vi "Shift Master.vi"(8 "error in (no error)":errorcluster) -> (0 "error out":errorcluster)   [LabVIEW 2017]
uses:
  <vilib>/Utility/miscctls.llb/LVRowAndColumnTypeDef.ctl
  <vilib>/Utility/miscctls.llb/LVBoundsTypeDef.ctl
  <vilib>/addons/database/Connection.llb/DB Tools Open Connec (Path).vi
  Globle/Current date.vi
  <vilib>/addons/database/NI_Database_API.lvlib
panel:
  in  "Back 2":bool
  in  "UPDATE   2":bool
  in  "MANUALLY":bool
  in  "12 HR SHIFT IN 24 HR FORMATE":bool
  in  "8 HR SHIFT IN 24 HR FORMATE":bool
  in  "Shift 3 Stop Time":timestamp format="%<%H-%M-%S>T"
  in  "Shift 2Stop Time":timestamp format="%<%H:%M:%S>T"
  in  "Shift 3 Start Time":timestamp format="%<%H-%M-%S>T"
  in  "Shift 2 Start Time":timestamp format="%<%H:%M:%S>T"
  in  "Shift 1 Stop Time":timestamp=timestamp(-9561628800 s since 1904-01-01) format="%<%H:%M:%S>T"
  in  "Shift 1 Start time":timestamp=timestamp(-9561628800 s since 1904-01-01) format="%<%H:%M:%S>T"
  # "Shift Master"
  # "Shift Start Time"
  # "Shift End Time"
  # "Shift Name"
  # "Shift One"
  # "Shift Two"
  # "Shift Three"
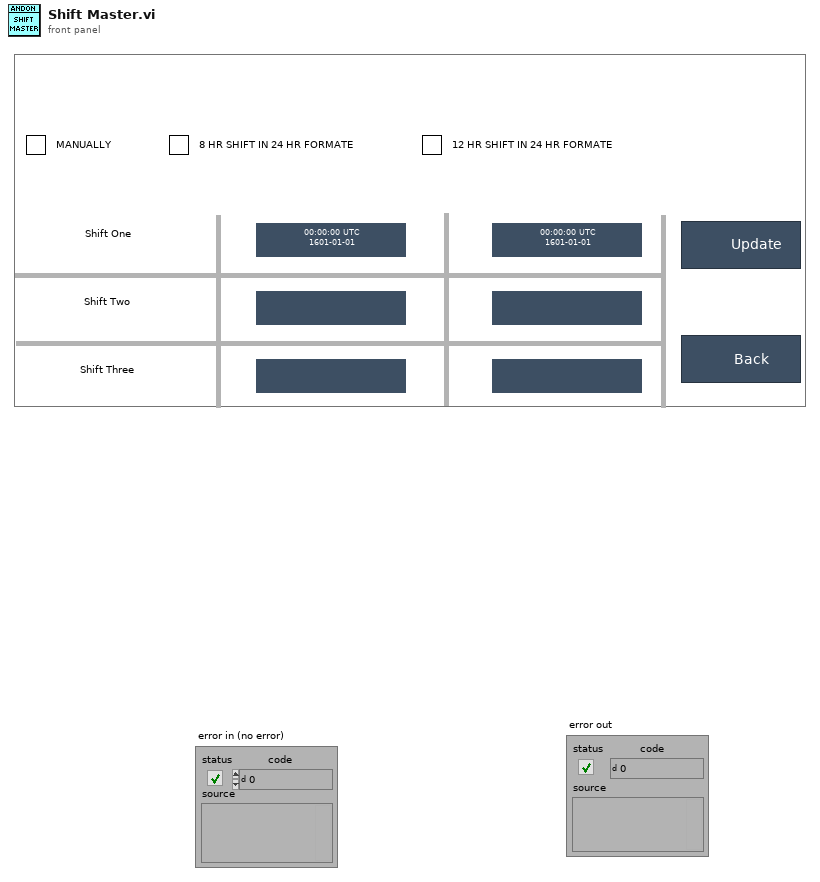
[diagram p1: front panel]
types:
  T1 = typedef "LVBoundsTypeDef.ctl" = cluster{"Width":u32, "Height":u32}
  T2 = typedef "LVRowAndColumnTypeDef.ctl" = cluster{"Row":i32, "Column":i32}
  T3 = enum8{"Enabled", "Disabled", "Disabled and Grayed Out"}
  T4 = typedef "NI_Database_API.lvlib/Conn ObjectReference.ctl" = refnum<k1>
  T5 = cluster{"Shift 3 Start Time":timestamp, "Shift 3 Stop Time ":timestamp}
  T6 = cluster{"Shift 2 Start Time":timestamp, "Shift 2Stop Time":timestamp}
  T7 = cluster{"Shift 1 Start time":timestamp, "Shift 1 Stop Time":timestamp}
  T8 = cluster{"Shift 3 Start Time":timestamp, "Shift 3 Stop Time ":timestamp}[]
  T9 = enum32{"invalid app kind", "Development System", "Run Time System", "Student Edition", "Embedded LabVIEW", "Evaluation", "Custom"}
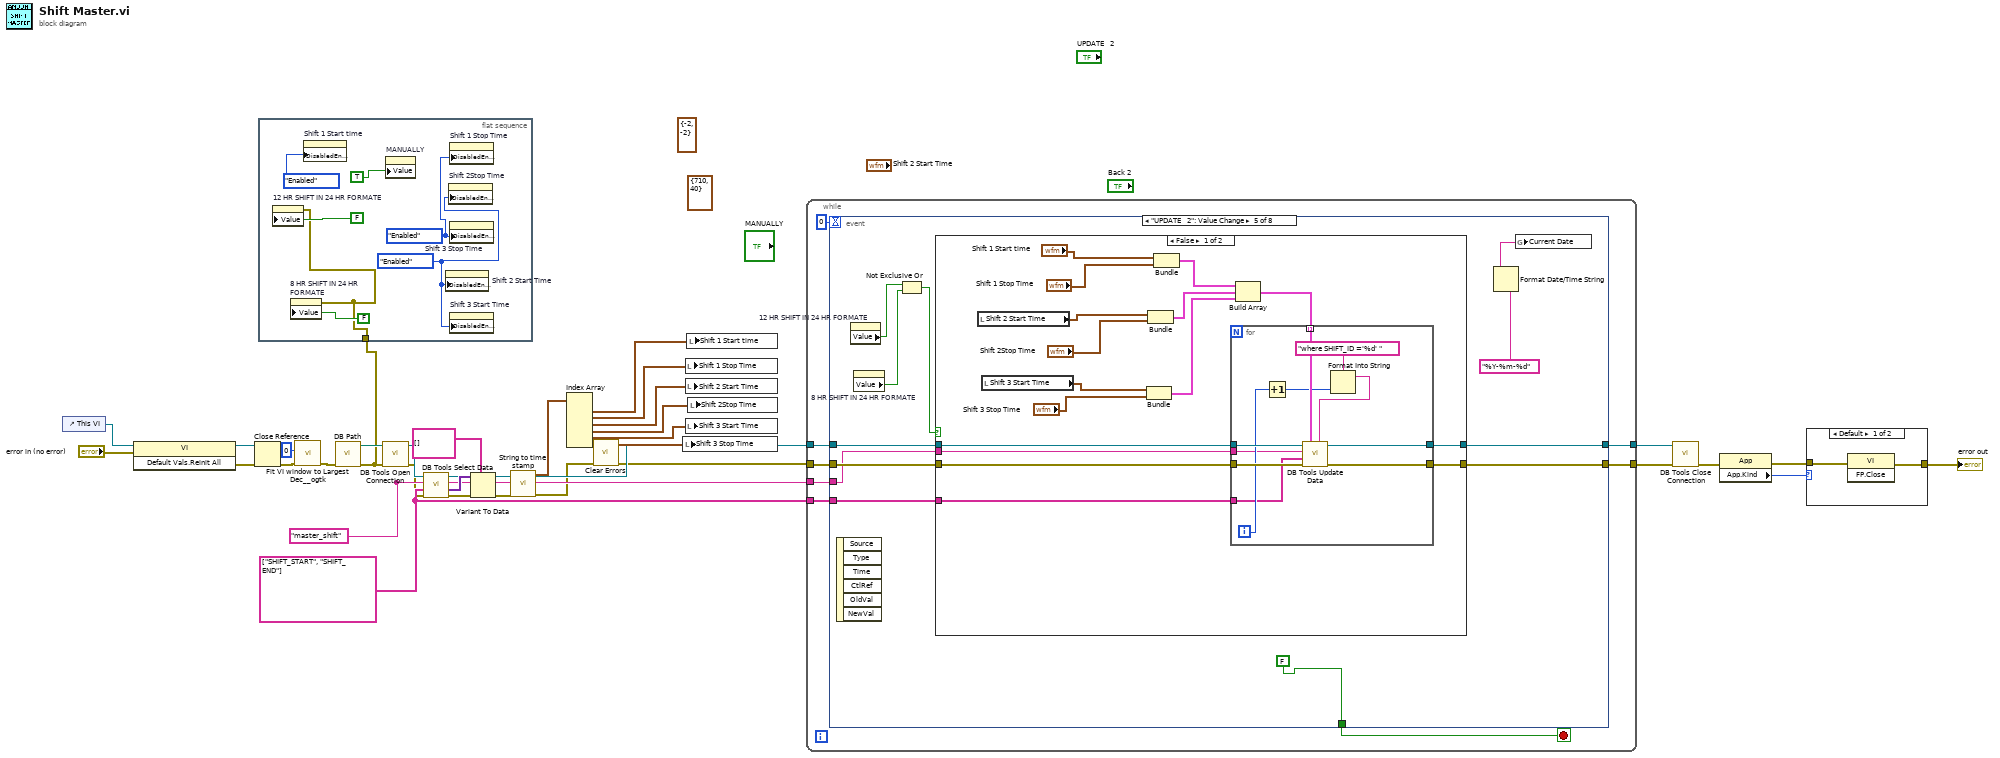
[diagram p0: block diagram]
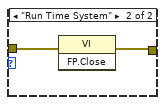
[diagram p2: hidden frame]
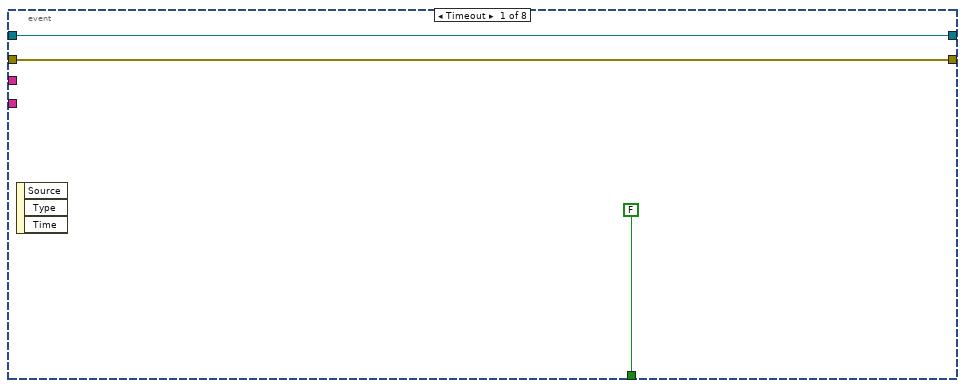
[diagram p3: hidden frame]
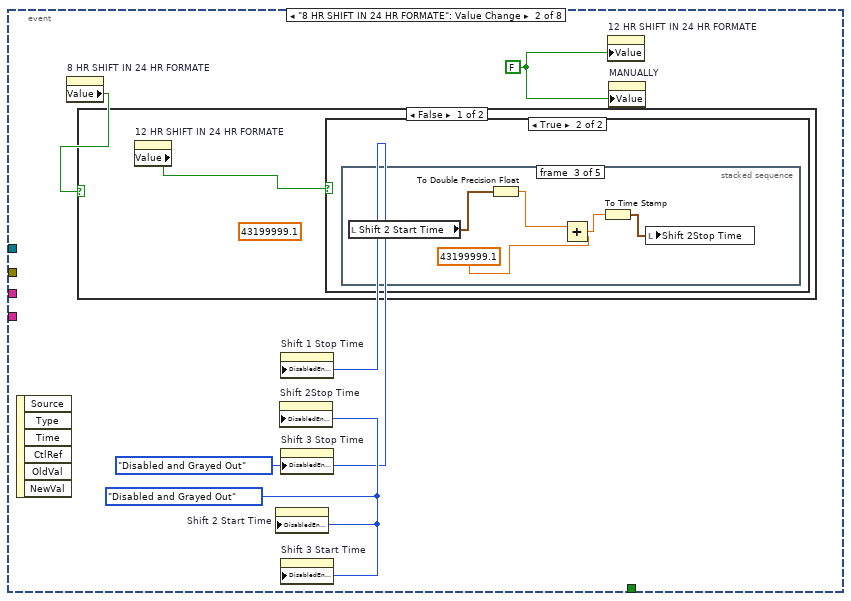
[diagram p4: hidden frame]
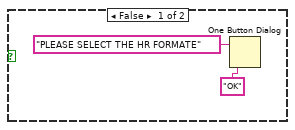
[diagram p5: hidden frame]
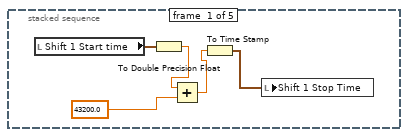
[diagram p6: hidden frame]
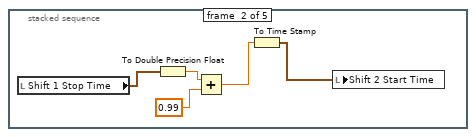
[diagram p7: hidden frame]
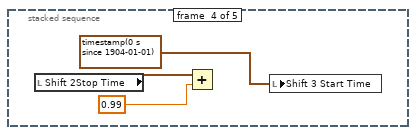
[diagram p8: hidden frame]
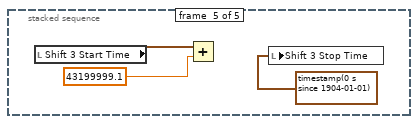
[diagram p9: hidden frame]
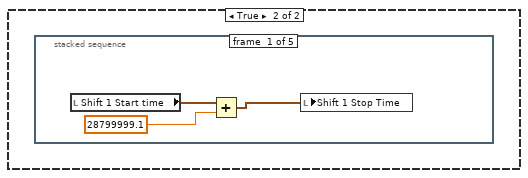
[diagram p10: hidden frame]
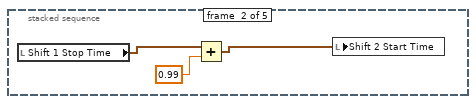
[diagram p11: hidden frame]
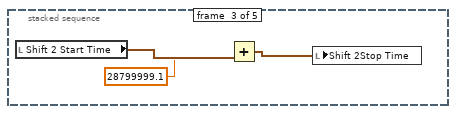
[diagram p12: hidden frame]
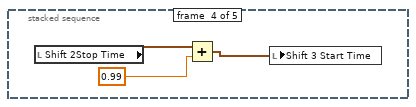
[diagram p13: hidden frame]
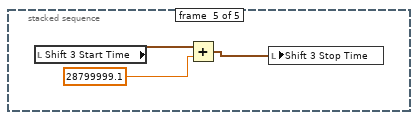
[diagram p14: hidden frame]
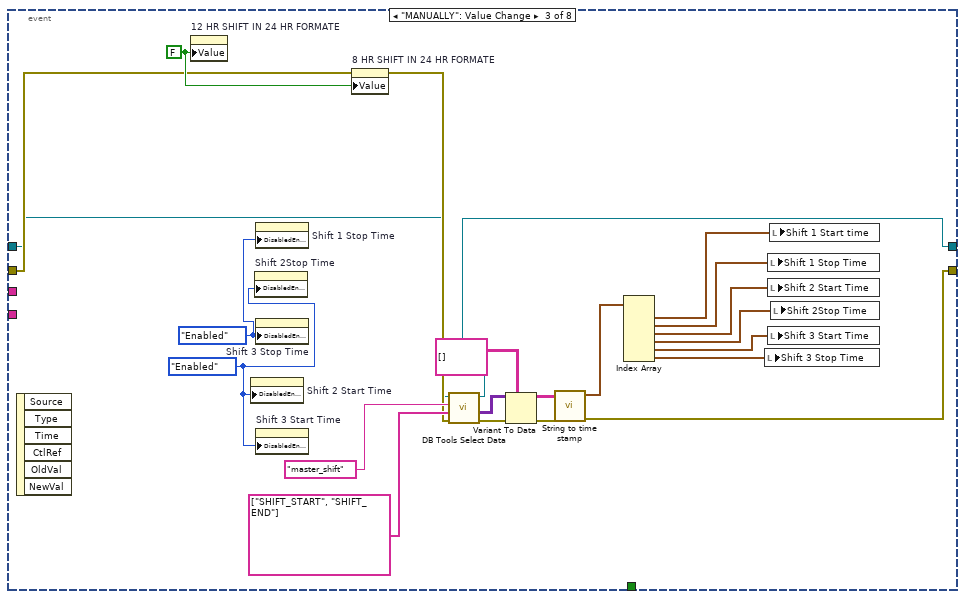
[diagram p15: hidden frame]
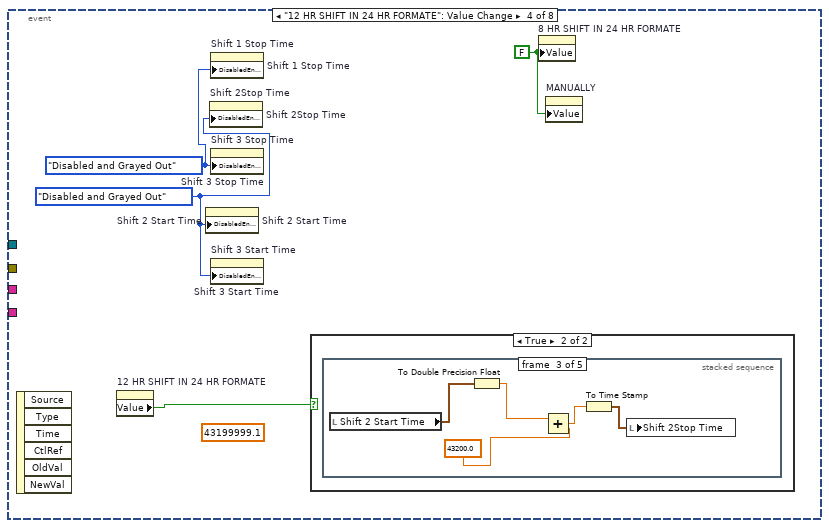
[diagram p16: hidden frame]
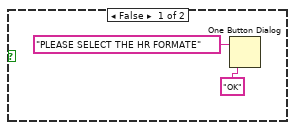
[diagram p17: hidden frame]
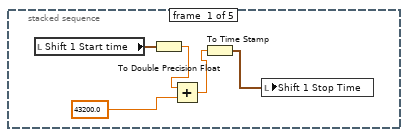
[diagram p18: hidden frame]
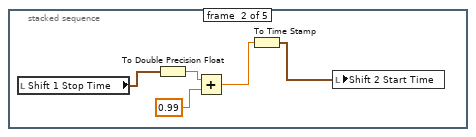
[diagram p19: hidden frame]
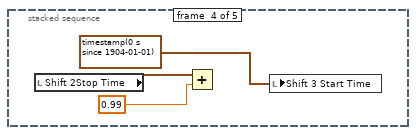
[diagram p20: hidden frame]
diagram:
  w10 = string[] ["SHIFT_START", "SHIFT_END"] ("columns")
  w11 = "master_shift" ("table")
  (unwired) T1 {"Width"=710, "Height"=40} ("Active Cell:Cell Size")
  (unwired) T2 {"Row"=-2, "Column"=-2} ("Active Cell:Active Cell")
  n1 = control-ref of="This VI"() -> (w34:refnum<vi>)
  n2 = invoke class="VI" method="Default Vals.Reinit All"(reference=w34, error in="error in (no error)") -> (reference out=w31:refnum<vi>, error out=w32:errorcluster)  [unwired: 1 in, 1 out]
  n3 = Close Reference(reference=w31, error in (no error)=w32) -> (error out=w4:errorcluster)
  n4 = flat-sequence {
    tunnel: w1 -> [w36]
    frame #0 {
      w41 = T3."Enabled" ("Disabled")
      w40 = T3."Enabled" ("Disabled")
      n5 = property on="12 HR SHIFT IN 24 HR FORMATE" class="Bool (strict)"(error in=w36, "Value"=FALSE ("12 HR FORMATE")) -> ()  [unwired: 1 in, 2 out]
      n6 = property on="8 HR SHIFT IN 24 HR FORMATE" class="Bool (strict)"(error in=w36, "Value"=FALSE ("8 HR FORMATE")) -> ()  [unwired: 1 in, 2 out]
      n7 = property on="Shift 1 Start time" class="AbsTime (strict)"("DisabledEnum"=T3."Enabled" ("Disabled")) -> ()  [unwired: 2 in, 2 out]
      n8 = property on="MANUALLY" class="Bool (strict)"("Value"=TRUE ("12 HR FORMATE")) -> ()  [unwired: 2 in, 2 out]
      n9 = property on="Shift 2 Start Time" class="AbsTime (strict)"("DisabledEnum"=w41) -> ()  [unwired: 2 in, 2 out]
      n10 = property on="Shift 2Stop Time" class="AbsTime (strict)"("DisabledEnum"=w41) -> ()  [unwired: 2 in, 2 out]
      n11 = property on="Shift 1 Stop Time" class="AbsTime (strict)"("DisabledEnum"=w40) -> ()  [unwired: 2 in, 2 out]
      n12 = property on="Shift 3 Stop Time" class="AbsTime (strict)"("DisabledEnum"=w40) -> ()  [unwired: 2 in, 2 out]
      n13 = property on="Shift 3 Start Time" class="AbsTime (strict)"("DisabledEnum"=w41) -> ()  [unwired: 2 in, 2 out]
    }
  }
  n14 = call <userlib>:"Fit VI window to Largest Dec__ogtk.vi"("error in (no error)"=w4, "border spacing (2 px)"=0) -> ("error out"=w3:errorcluster)  [unwired: 4 in, 1 out]
  n15 = call "DB Path.vi"("error in"=w3) -> ("error out"=w1:errorcluster, "DB Path"=w27:path)  [unwired: 9 in]
  n16 = call-poly <vilib>:"DB Tools Open Connection.vi"("error in (no error)"=w1, "connection information"=w27) -> ("error out"=w5:errorcluster, "connection reference"=w6:T4)  [unwired: 6 in]
  n17 = call <vilib>:"DB Tools Select Data.vi"("error in (no error)"=w5, "columns"=w10, "table"=w11, "connection reference"=w6) -> ("error out"=w25:errorcluster, "data"=w26:variant[][], "connection reference out"=w15:T4)  [unwired: 2 in]
  n18 = Variant To Data(error in=w25, type=string[][] [], Variant=w26) -> (data=w9:string[][], error out=w23:errorcluster)
  n19 = call "String to time stamp.vi"("error in (no error)"=w23, "Data In"=w9) -> ("error out"=w8:errorcluster, "Time Stamp Out"=w22:timestamp[])  [unwired: 8 in]
  n20 = Index Array(array=w22) -> (element #1=w21:timestamp, element #2=w20:timestamp, element #3=w19:timestamp, element #4=w18:timestamp, element #5=w17:timestamp, element #6=w16:timestamp)  [unwired: 6 in]
  n21 = call <vilib>:"Clear Errors.vi"("error in (no error)"=w8) -> ("error out"=w7:errorcluster)  [unwired: 5 in, 1 out]
  n22 = local write "Shift 3 Stop Time"(w16) -> ()
  n23 = local write "Shift 1 Stop Time"(w20) -> ()
  n24 = local write "Shift 2 Start Time"(w19) -> ()
  n25 = local write "Shift 3 Start Time"(w17) -> ()
  n26 = local write "Shift 1 Start time"(w21) -> ()
  n27 = local write "Shift 2Stop Time"(w18) -> ()
  n28 = while {
    tunnel: w7 -> [w49]
    tunnel: [w47] -> w14
    tunnel: w15 -> [w46]
    tunnel: [w45] -> w12
    tunnel: w11 -> [w44]
    tunnel: w10 -> [w43]
    stop <- w48 stop-if-true
    n29 = event shown="[4] \"UPDATE   2\": Value Change" {
      selector: _ -> [_ _ _ _ _ _ _ _]
      dyn-events: _ -> [_ _ _ _ _ _ _ _]
      timeout: 0 -> [_ _ _ _ _ _ _ _]
      tunnel: w49 -> [w51 _ w99 _ w158 w191 w193 w200]
      tunnel: [FALSE _ _ _ FALSE TRUE _ FALSE] -> w48
      tunnel: [w51 _ w98 _ w154 w191 w193 w200] -> w47
      tunnel: w46 -> [w52 _ w97 _ w157 w192 _ w198]
      tunnel: [w52 _ w96 _ w153 w192 _ w198] -> w45
      tunnel: w44 -> [_ _ _ _ w156 _ _ _]
      tunnel: w43 -> [_ _ _ _ w155 _ _ _]
      event Timeout {
        n30 = event-data() -> ()  [unwired: 1 in, 3 out]
      }
      event "8 HR SHIFT IN 24 HR FORMATE": Value Change {
        w54 = T3."Disabled and Grayed Out" ("Disabled")
        w53 = T3."Disabled and Grayed Out" ("Disabled")
        w55 = FALSE ("12 HR FORMATE")
        n31 = event-data() -> ()  [unwired: 1 in, 6 out]
        n32 = property on="8 HR SHIFT IN 24 HR FORMATE" class="Bool (strict)"() -> ("Value"=w56:bool)  [unwired: 2 in, 2 out]
        n33 = case shown="False" w56 {
          frame False {
            (unwired) 43199999.1 ("y")
            n34 = property on="12 HR SHIFT IN 24 HR FORMATE" class="Bool (strict)"() -> ("Value"=w57:bool)  [unwired: 2 in, 2 out]
            n35 = case shown="True" w57 {
              frame False {
                n36 = One Button Dialog(message="PLEASE SELECT THE HR FORMATE", button name ("OK")="OK") -> ()  [unwired: 1 out]
              }
              frame True {
                n37 = stacked-sequence {
                  frame #0 {
                    n38 = local read "Shift 1 Start time"() -> (w63:timestamp)
                    n39 = To Double Precision Float(number=w63) -> (double precision float=w62:dbl)
                    n40 = Add(x=w62, y=43200.0) -> (x+y=w61:dbl)
                    n41 = To Time Stamp(1:w61) -> (0:w60:timestamp)
                    n42 = local write "Shift 1 Stop Time"(w60) -> ()
                  }
                  frame #1 {
                    n43 = local read "Shift 1 Stop Time"() -> (w66:timestamp)
                    n44 = To Double Precision Float(number=w66) -> (double precision float=w65:dbl)
                    n45 = Add(x=w65, y=0.99) -> (x+y=w67:dbl)
                    n46 = To Time Stamp(1:w67) -> (0:w68:timestamp)
                    n47 = local write "Shift 2 Start Time"(w68) -> ()
                  }
                  frame #2 {
                    n48 = local read "Shift 2 Start Time"() -> (w71:timestamp)
                    n49 = To Double Precision Float(number=w71) -> (double precision float=w70:dbl)
                    n50 = Add(x=w70, y=43199999.1) -> (x+y=w73:dbl)
                    n51 = To Time Stamp(1:w73) -> (0:w72:timestamp)
                    n52 = local write "Shift 2Stop Time"(w72) -> ()
                  }
                  frame #3 {
                    n53 = local read "Shift 2Stop Time"() -> (w77:timestamp)
                    n54 = Add(x=w77, y=0.99) -> ()  [unwired: 1 out]
                    n55 = local write "Shift 3 Start Time"(timestamp(0 s since 1904-01-01) ("x+y")) -> ()
                  }
                  frame #4 {
                    n56 = local read "Shift 3 Start Time"() -> (w80:timestamp)
                    n57 = Add(x=w80, y=43199999.1) -> ()  [unwired: 1 out]
                    n58 = local write "Shift 3 Stop Time"(timestamp(0 s since 1904-01-01) ("x+y")) -> ()
                  }
                }
              }
            }
          }
          frame True {
            n59 = stacked-sequence {
              frame #0 {
                n60 = local read "Shift 1 Start time"() -> (w83:timestamp)
                n61 = Add(x=w83, y=28799999.1) -> (x+y=w81:timestamp)
                n62 = local write "Shift 1 Stop Time"(w81) -> ()
              }
              frame #1 {
                n63 = local read "Shift 1 Stop Time"() -> (w84:timestamp)
                n64 = Add(x=w84, y=0.99) -> (x+y=w86:timestamp)
                n65 = local write "Shift 2 Start Time"(w86) -> ()
              }
              frame #2 {
                n66 = local read "Shift 2 Start Time"() -> (w89:timestamp)
                n67 = Add(x=w89, y=28799999.1) -> (x+y=w88:timestamp)
                n68 = local write "Shift 2Stop Time"(w88) -> ()
              }
              frame #3 {
                n69 = local read "Shift 2Stop Time"() -> (w91:timestamp)
                n70 = Add(x=w91, y=0.99) -> (x+y=w92:timestamp)
                n71 = local write "Shift 3 Start Time"(w92) -> ()
              }
              frame #4 {
                n72 = local read "Shift 3 Start Time"() -> (w95:timestamp)
                n73 = Add(x=w95, y=28799999.1) -> (x+y=w94:timestamp)
                n74 = local write "Shift 3 Stop Time"(w94) -> ()
              }
            }
          }
        }
        n75 = property on="Shift 2 Start Time" class="AbsTime (strict)"("DisabledEnum"=w54) -> ()  [unwired: 2 in, 2 out]
        n76 = property on="Shift 2Stop Time" class="AbsTime (strict)"("DisabledEnum"=w54) -> ()  [unwired: 2 in, 2 out]
        n77 = property on="Shift 1 Stop Time" class="AbsTime (strict)"("DisabledEnum"=w53) -> ()  [unwired: 2 in, 2 out]
        n78 = property on="Shift 3 Stop Time" class="AbsTime (strict)"("DisabledEnum"=w53) -> ()  [unwired: 2 in, 2 out]
        n79 = property on="Shift 3 Start Time" class="AbsTime (strict)"("DisabledEnum"=w54) -> ()  [unwired: 2 in, 2 out]
        n80 = property on="12 HR SHIFT IN 24 HR FORMATE" class="Bool (strict)"("Value"=w55) -> ()  [unwired: 2 in, 2 out]
        n81 = property on="MANUALLY" class="Bool (strict)"("Value"=w55) -> ()  [unwired: 2 in, 2 out]
      }
      event "MANUALLY": Value Change {
        w115 = FALSE ("12 HR SHIFT IN 24 HR FORMATE")
        w117 = T3."Enabled" ("Disabled")
        w116 = T3."Enabled" ("Disabled")
        n82 = event-data() -> ()  [unwired: 1 in, 6 out]
        n83 = property on="12 HR SHIFT IN 24 HR FORMATE" class="Bool (strict)"("Value"=w115) -> ()  [unwired: 2 in, 2 out]
        n84 = property on="Shift 2 Start Time" class="AbsTime (strict)"("DisabledEnum"=w117) -> ()  [unwired: 2 in, 2 out]
        n85 = property on="Shift 2Stop Time" class="AbsTime (strict)"("DisabledEnum"=w117) -> ()  [unwired: 2 in, 2 out]
        n86 = property on="Shift 1 Stop Time" class="AbsTime (strict)"("DisabledEnum"=w116) -> ()  [unwired: 2 in, 2 out]
        n87 = property on="Shift 3 Stop Time" class="AbsTime (strict)"("DisabledEnum"=w116) -> ()  [unwired: 2 in, 2 out]
        n88 = property on="Shift 3 Start Time" class="AbsTime (strict)"("DisabledEnum"=w117) -> ()  [unwired: 2 in, 2 out]
        n89 = property on="8 HR SHIFT IN 24 HR FORMATE" class="Bool (strict)"(error in=w99, "Value"=w115) -> (error out=w100:errorcluster)  [unwired: 1 in, 1 out]
        n90 = call <vilib>:"DB Tools Select Data.vi"("error in (no error)"=w100, "columns"=string[] ["SHIFT_START", "SHIFT_END"], "table"="master_shift", "connection reference"=w97) -> ("error out"=w113:errorcluster, "data"=w114:variant[][], "connection reference out"=w96:T4)  [unwired: 2 in]
        n91 = Variant To Data(error in=w113, type=string[][] [], Variant=w114) -> (data=w104:string[][], error out=w112:errorcluster)
        n92 = call "String to time stamp.vi"("error in (no error)"=w112, "Data In"=w104) -> ("error out"=w98:errorcluster, "Time Stamp Out"=w111:timestamp[])  [unwired: 8 in]
        n93 = Index Array(array=w111) -> (element #1=w110:timestamp, element #2=w109:timestamp, element #3=w108:timestamp, element #4=w107:timestamp, element #5=w106:timestamp, element #6=w105:timestamp)  [unwired: 6 in]
        n94 = local write "Shift 3 Stop Time"(w105) -> ()
        n95 = local write "Shift 1 Stop Time"(w109) -> ()
        n96 = local write "Shift 2 Start Time"(w108) -> ()
        n97 = local write "Shift 3 Start Time"(w106) -> ()
        n98 = local write "Shift 1 Start time"(w110) -> ()
        n99 = local write "Shift 2Stop Time"(w107) -> ()
      }
      event "12 HR SHIFT IN 24 HR FORMATE": Value Change {
        w119 = T3."Disabled and Grayed Out" ("Disabled")
        w118 = T3."Disabled and Grayed Out" ("Disabled")
        w120 = T3."Disabled and Grayed Out" ("Disabled")
        w121 = T3."Disabled and Grayed Out" ("Disabled")
        (unwired) 43199999.1 ("y")
        w122 = FALSE ("8 HR FORMATE")
        n100 = event-data() -> ()  [unwired: 1 in, 6 out]
        n101 = property on="12 HR SHIFT IN 24 HR FORMATE" class="Bool (strict)"() -> ("Value"=w123:bool)  [unwired: 2 in, 2 out]
        n102 = property on="Shift 2 Start Time" class="AbsTime (strict)"("DisabledEnum"=w119) -> ()  [unwired: 2 in, 2 out]
        n103 = property on="Shift 2 Start Time" class="AbsTime (strict)"("DisabledEnum"=w120) -> ()  [unwired: 2 in, 2 out]
        n104 = property on="Shift 2Stop Time" class="AbsTime (strict)"("DisabledEnum"=w119) -> ()  [unwired: 2 in, 2 out]
        n105 = property on="Shift 2Stop Time" class="AbsTime (strict)"("DisabledEnum"=w120) -> ()  [unwired: 2 in, 2 out]
        n106 = property on="Shift 1 Stop Time" class="AbsTime (strict)"("DisabledEnum"=w118) -> ()  [unwired: 2 in, 2 out]
        n107 = property on="Shift 1 Stop Time" class="AbsTime (strict)"("DisabledEnum"=w121) -> ()  [unwired: 2 in, 2 out]
        n108 = property on="Shift 3 Stop Time" class="AbsTime (strict)"("DisabledEnum"=w118) -> ()  [unwired: 2 in, 2 out]
        n109 = property on="Shift 3 Stop Time" class="AbsTime (strict)"("DisabledEnum"=w121) -> ()  [unwired: 2 in, 2 out]
        n110 = property on="Shift 3 Start Time" class="AbsTime (strict)"("DisabledEnum"=w119) -> ()  [unwired: 2 in, 2 out]
        n111 = property on="Shift 3 Start Time" class="AbsTime (strict)"("DisabledEnum"=w120) -> ()  [unwired: 2 in, 2 out]
        n112 = case shown="True" w123 {
          frame False {
            n113 = One Button Dialog(message="PLEASE SELECT THE HR FORMATE", button name ("OK")="OK") -> ()  [unwired: 1 out]
          }
          frame True {
            n114 = stacked-sequence {
              frame #0 {
                n115 = local read "Shift 1 Start time"() -> (w129:timestamp)
                n116 = To Double Precision Float(number=w129) -> (double precision float=w128:dbl)
                n117 = Add(x=w128, y=43200.0) -> (x+y=w127:dbl)
                n118 = To Time Stamp(1:w127) -> (0:w126:timestamp)
                n119 = local write "Shift 1 Stop Time"(w126) -> ()
              }
              frame #1 {
                n120 = local read "Shift 1 Stop Time"() -> (w132:timestamp)
                n121 = To Double Precision Float(number=w132) -> (double precision float=w131:dbl)
                n122 = Add(x=w131, y=0.99) -> (x+y=w133:dbl)
                n123 = To Time Stamp(1:w133) -> (0:w134:timestamp)
                n124 = local write "Shift 2 Start Time"(w134) -> ()
              }
              frame #2 {
                n125 = local read "Shift 2 Start Time"() -> (w137:timestamp)
                n126 = To Double Precision Float(number=w137) -> (double precision float=w136:dbl)
                n127 = Add(x=w136, y=43200.0) -> (x+y=w139:dbl)
                n128 = To Time Stamp(1:w139) -> (0:w138:timestamp)
                n129 = local write "Shift 2Stop Time"(w138) -> ()
              }
              frame #3 {
                n130 = local read "Shift 2Stop Time"() -> (w143:timestamp)
                n131 = Add(x=w143, y=0.99) -> ()  [unwired: 1 out]
                n132 = local write "Shift 3 Start Time"(timestamp(0 s since 1904-01-01) ("x+y")) -> ()
              }
              frame #4 {
                n133 = local read "Shift 3 Start Time"() -> (w146:timestamp)
                n134 = Add(x=w146, y=43199999.1) -> ()  [unwired: 1 out]
                n135 = local write "Shift 3 Stop Time"(timestamp(0 s since 1904-01-01) ("x+y")) -> ()
              }
            }
          }
        }
        n136 = property on="8 HR SHIFT IN 24 HR FORMATE" class="Bool (strict)"("Value"=w122) -> ()  [unwired: 2 in, 2 out]
        n137 = property on="MANUALLY" class="Bool (strict)"("Value"=w122) -> ()  [unwired: 2 in, 2 out]
      }
      event "UPDATE   2": Value Change {
        n138 = event-data() -> ()  [unwired: 1 in, 6 out]
        n139 = property on="12 HR SHIFT IN 24 HR FORMATE" class="Bool (strict)"() -> ("Value"=w150:bool)  [unwired: 2 in, 2 out]
        n140 = property on="8 HR SHIFT IN 24 HR FORMATE" class="Bool (strict)"() -> ("Value"=w149:bool)  [unwired: 2 in, 2 out]
        n141 = Not Exclusive Or(1:w149, 2:w150) -> (0:w148:bool)
        n142 = case shown="False" w148 {
          tunnel: w158 -> [w166 w186]
          tunnel: w157 -> [w165 w187]
          tunnel: w156 -> [w164 _]
          tunnel: w155 -> [w163 _]
          tunnel: [w160 w186] -> w154
          tunnel: [w159 w187] -> w153
          frame False {
            n143 = local read "Shift 2 Start Time"() -> (w171:timestamp)
            n144 = local read "Shift 3 Start Time"() -> (w170:timestamp)
            n145 = Bundle("Shift 3 Start Time"=w170, "Shift 3 Stop Time"="Shift 3 Stop Time") -> (w168:T5)  [unwired: 1 in]
            n146 = Bundle("Shift 2 Start Time"=w171, "Shift 2Stop Time"="Shift 2Stop Time") -> (w169:T6)  [unwired: 1 in]
            n147 = Bundle("Shift 1 Start time"="Shift 1 Start time", "Shift 1 Stop Time"="Shift 1 Stop Time") -> (w167:T7)  [unwired: 1 in]
            n148 = Build Array(w167, w169, w168) -> (w162:T8)
            n149 = for {
              tunnel: w164 -> [w175]
              tunnel: w163 -> [w176]
              tunnel: w162 -> [w181] mode=indexing
              tunnel: w165 -> [w183]
              tunnel: [w182] -> w159
              tunnel: w166 -> [w185]
              tunnel: [w184] -> w160
              i -> [w178]
              n150 = Increment(x=w178) -> (x+1=w177:i32)
              n151 = Format Into String(format string="where SHIFT_ID ='%d' ", w177) -> (resulting string=w180:string)  [unwired: 2 in, 1 out]
              n152 = call <vilib>:"DB Tools Update Data.vi"("condition"=w180, "data"=w181, "error in (no error)"=w185, "columns"=w176, "table"=w175, "connection reference"=w183) -> ("error out"=w184:errorcluster, "connection reference out"=w182:T4)  [unwired: 4 in]
            }
          }
          frame True {
            n153 = One Button Dialog(message="PLEASE SELECT THE HR FORMATE", button name ("OK")="OK") -> ()  [unwired: 1 out]
          }
        }
        n154 = Format Date/Time String(time format string (%c)="%Y-%m-%d") -> (date/time string=w152:string)  [unwired: 2 in]
        n155 = global write "Current date.vi" "Current Date"(w152) -> ()
      }
      event "Back 2": Value Change {
        n156 = event-data() -> ()  [unwired: 1 in, 6 out]
      }
      event "Shift 2Stop Time": Value Change {
        n157 = event-data() -> ()  [unwired: 1 in, 6 out]
        n158 = disable-structure shown="Disabled" {
          frame Disabled {
            n159 = local read "Shift 2Stop Time"() -> (w196:timestamp)
            n160 = Add(x=w196, y=1.0) -> (x+y=w194:timestamp)
            n161 = local write "Shift 3 Start Time"(w194) -> ()
          }
          frame Enabled {
          }
        }
      }
      event "Shift 1 Start time": Value Change {
        n162 = event-data() -> ()  [unwired: 1 in, 6 out]
        n163 = case shown="False" "8 HR SHIFT IN 24 HR FORMATE" {
          frame False {
            (unwired) 43199999.1 ("y")
            n164 = case shown="True" "12 HR SHIFT IN 24 HR FORMATE" {
              frame False {
                n165 = One Button Dialog(message="PLEASE SELECT THE HR FORMATE", button name ("OK")="OK") -> ()  [unwired: 1 out]
              }
              frame True {
                n166 = stacked-sequence {
                  frame #0 {
                    n167 = local read "Shift 1 Start time"() -> (w207:timestamp)
                    n168 = To Double Precision Float(number=w207) -> (double precision float=w206:dbl)
                    n169 = Add(x=w206, y=43200.0) -> (x+y=w205:dbl)
                    n170 = To Time Stamp(1:w205) -> (0:w204:timestamp)
                    n171 = local write "Shift 1 Stop Time"(w204) -> ()
                  }
                  frame #1 {
                    n172 = local read "Shift 1 Stop Time"() -> (w210:timestamp)
                    n173 = To Double Precision Float(number=w210) -> (double precision float=w209:dbl)
                    n174 = Add(x=w209, y=0.99) -> (x+y=w211:dbl)
                    n175 = To Time Stamp(1:w211) -> (0:w212:timestamp)
                    n176 = local write "Shift 2 Start Time"(w212) -> ()
                  }
                  frame #2 {
                    n177 = local read "Shift 2 Start Time"() -> (w215:timestamp)
                    n178 = To Double Precision Float(number=w215) -> (double precision float=w214:dbl)
                    n179 = Add(x=w214, y=43200.0) -> (x+y=w217:dbl)
                    n180 = To Time Stamp(1:w217) -> (0:w216:timestamp)
                    n181 = local write "Shift 2Stop Time"(w216) -> ()
                  }
                  frame #3 {
                    n182 = local read "Shift 2Stop Time"() -> (w221:timestamp)
                    n183 = Add(x=w221, y=0.99) -> ()  [unwired: 1 out]
                    n184 = local write "Shift 3 Start Time"(timestamp(0 s since 1904-01-01) ("x+y")) -> ()
                  }
                  frame #4 {
                    n185 = local read "Shift 3 Start Time"() -> (w224:timestamp)
                    n186 = Add(x=w224, y=43199999.1) -> ()  [unwired: 1 out]
                    n187 = local write "Shift 3 Stop Time"(timestamp(0 s since 1904-01-01) ("x+y")) -> ()
                  }
                }
              }
            }
          }
          frame True {
            n188 = stacked-sequence {
              frame #0 {
                n189 = local read "Shift 1 Start time"() -> (w227:timestamp)
                n190 = Add(x=w227, y=28799999.1) -> (x+y=w225:timestamp)
                n191 = local write "Shift 1 Stop Time"(w225) -> ()
              }
              frame #1 {
                n192 = local read "Shift 1 Stop Time"() -> (w228:timestamp)
                n193 = Add(x=w228, y=0.99) -> (x+y=w230:timestamp)
                n194 = local write "Shift 2 Start Time"(w230) -> ()
              }
              frame #2 {
                n195 = local read "Shift 2 Start Time"() -> (w233:timestamp)
                n196 = Add(x=w233, y=28799999.1) -> (x+y=w232:timestamp)
                n197 = local write "Shift 2Stop Time"(w232) -> ()
              }
              frame #3 {
                n198 = local read "Shift 2Stop Time"() -> (w235:timestamp)
                n199 = Add(x=w235, y=0.99) -> (x+y=w236:timestamp)
                n200 = local write "Shift 3 Start Time"(w236) -> ()
              }
              frame #4 {
                n201 = local read "Shift 3 Start Time"() -> (w239:timestamp)
                n202 = Add(x=w239, y=28799999.1) -> (x+y=w238:timestamp)
                n203 = local write "Shift 3 Stop Time"(w238) -> ()
              }
            }
          }
        }
      }
    }
  }
  n204 = call <vilib>:"DB Tools Close Connection.vi"("error in (no error)"=w14, "connection reference"=w12) -> ("error out"=w13:errorcluster)  [unwired: 5 in]
  n205 = property class="App"(error in=w13) -> (error out=w29:errorcluster, "App.Kind"=w30:T9)  [unwired: 1 in, 1 out]
  n206 = case shown="Default" w30 {
    tunnel: w29 -> [w241 w243]
    tunnel: [w240 w242] -> w28
    frame Default {
      n207 = invoke class="VI" method="FP.Close"(error in=w241) -> (error out=w240:errorcluster)  [unwired: 2 in, 2 out]
    }
    frame "Run Time System" {
      n208 = invoke class="VI" method="FP.Close"(error in=w243) -> (error out=w242:errorcluster)  [unwired: 2 in, 2 out]
    }
  }
  "error out" <- w28
